vi "Find IT6333A.vi"(8 "error in (no error)":errorcluster, 11 "PowerSupply_IT6333A in":refnum<class "PowerSupply_IT6333A.lvclass">) -> (0 "error out":errorcluster, 3 "PowerSupply_IT6333A out":refnum<class "PowerSupply_IT6333A.lvclass">)   [LabVIEW 2017, in "PowerSupply_IT6333A.lvclass"]
uses:
  PowerSupply_IT6333A.lvclass
  <vilib>/Instr/_visa.llb/VISA Find Search Mode.ctl
panel:
  out "find list":string[](array[string])
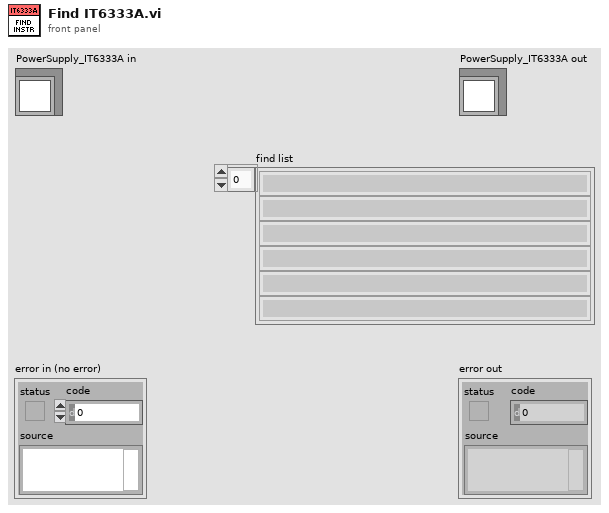
[diagram p1: front panel]
types:
  T1 = typedef "VISA Find Search Mode.ctl" = u32
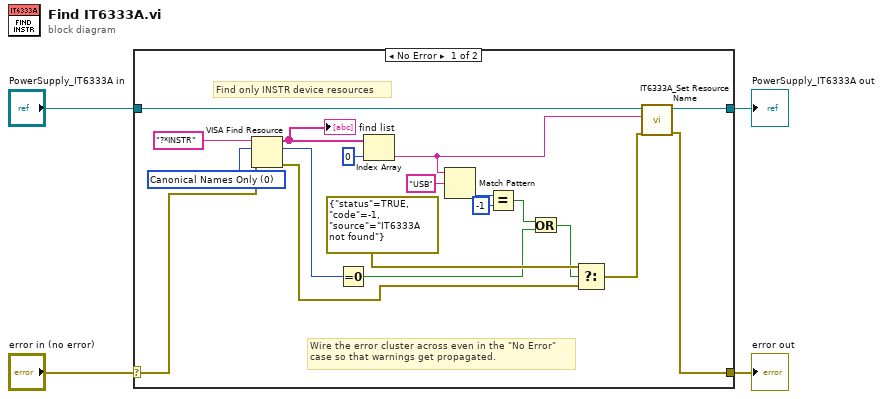
[diagram p0: block diagram]
diagram:
  n1 = case shown="No Error" "error in (no error)" {
    selector: "error in (no error)" -> [w13 w25]
    tunnel: [w12 w25] -> w3
    tunnel: [w22 w24] -> w1
    tunnel: "PowerSupply_IT6333A in" -> [w23 w24]
    frame No Error {
      w16 = T1 0 items=["Canonical Names Only"=0, "Aliases Only"=2, "Include Matching Aliases"=3, "Include All Aliases"=4] ("Search Mode")
      # "Find only INSTR device resources"
      # "Wire the error cluster across even in the \"No Error\"\ncase so that warnings get propagated."
      n2 = VISA Find Resource(8:w13, 10:w16, 11:"?*INSTR" ("expression (\"?*\")")) -> (0:w21:errorcluster, 2:w19:u32, 3:w17:string[])
      "find list" <- w17
      n3 = Equal To 0?(x=w19) -> (x = 0?=w6:bool)
      n4 = Index Array(array=w17, index=0) -> (element=w11:string)
      n5 = Match Pattern(string=w11, regular expression="USB") -> (offset past match=w9:i32)  [unwired: 1 in, 3 out]
      n6 = Equal?(x=w9, y=-1) -> (x = y?=w7:bool)
      n7 = Or(x=w7, y=w6) -> (x .or. y?=w5:bool)
      n8 = Select(t=errorcluster {"status"=TRUE, "code"=-1, "source"="IT6333A not found"} ("error constant"), s=w5, f=w21) -> (s? t:f=w14:errorcluster)
      n9 = call-dynamic "IT6333A_Set Resource Name.vi"("error in (no error)"=w14, "Resource Name"=w11, "PowerSupply_IT6333A in"=w23) -> ("error out"=w12:errorcluster, "PowerSupply_IT6333A out"=w22:refnum<class "PowerSupply_IT6333A.lvclass">)  [unwired: 7 in]
    }
    frame Error {
    }
  }
  "error out" <- w3
  "PowerSupply_IT6333A out" <- w1
